vi "doubles dash fg.vi"(1 "Shooter Bias":dbl, 2 "Menu":T1) -> (0 "Output":dbl)   [LabVIEW 2011]
uses:
  fg_typedef.ctl
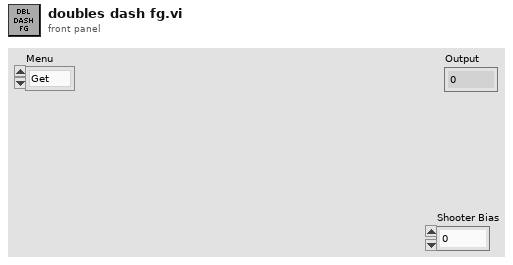
[diagram p1: front panel]
types:
  T1 = typedef "fg_typedef.ctl" = enum16{"Get", "Set"}
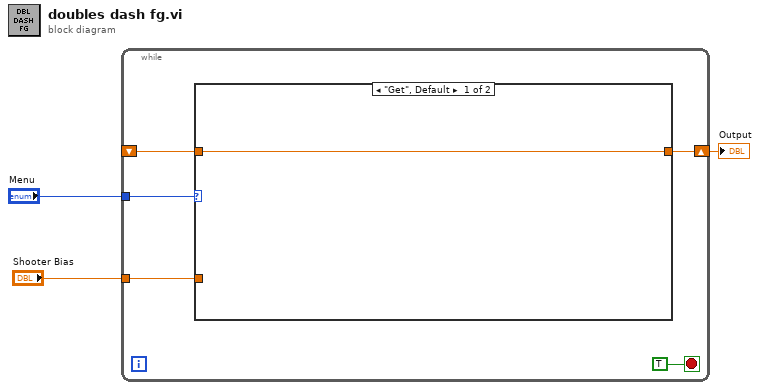
[diagram p0: block diagram]
diagram:
  n1 = while {
    tunnel: "Menu" -> [w7]
    tunnel: "Shooter Bias" -> [w6]
    shift-right: [w4] -> w1
    shift-left: _ -> [w5]
    stop <- TRUE stop-if-true
    n2 = case shown="\"Get\", Default" w7 {
      tunnel: w6 -> [_ w10]
      tunnel: w5 -> [w9 _]
      tunnel: [w9 w10] -> w4
      frame "Get", Default {
      }
      frame "Set" {
      }
    }
  }
  "Output" <- w1
